vi "calcualte_Vr_Vi.vi"(5 "C2":fxp<+/-,32,3>=0.002117181196808815 format="%#_30g", 7 "C1":fxp<+/-,32,3>=0.9986428320407867 format="%#_31g", 8 "input valid":bool=TRUE, 9 "dw*dt":fxp<+/-,48,0>, 10 "Ii":fxp<+/-,16,14>, 11 "Ir":fxp<+/-,16,14>) -> (0 "output valid":bool, 2 "Vi":fxp<+/-,48,16>, 3 "Vr":fxp<+/-,48,16>)   [LabVIEW 2013]
uses:
  <vilib>/rvi/FXPMathLib/FxpMul/XNode/nifxpmath_Multiplier.xnode
  <vilib>/rvi/FXPMathLib/FxpAdd/XNode/nifxpmath_Add.xnode
  <vilib>/rvi/FXPMathLib/FxpSub/XNode/nifxpmath_Sub.xnode
  <vilib>/rvi/FXPMathLib/sim/FxpSim.dll
panel:
  # "1-w12*dt = 0.998643"
  # "Rl*w12*dt*(10^-9) = 0.0021171821211066989"
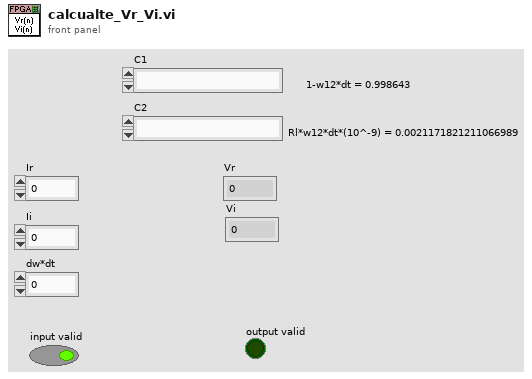
[diagram p1: front panel]
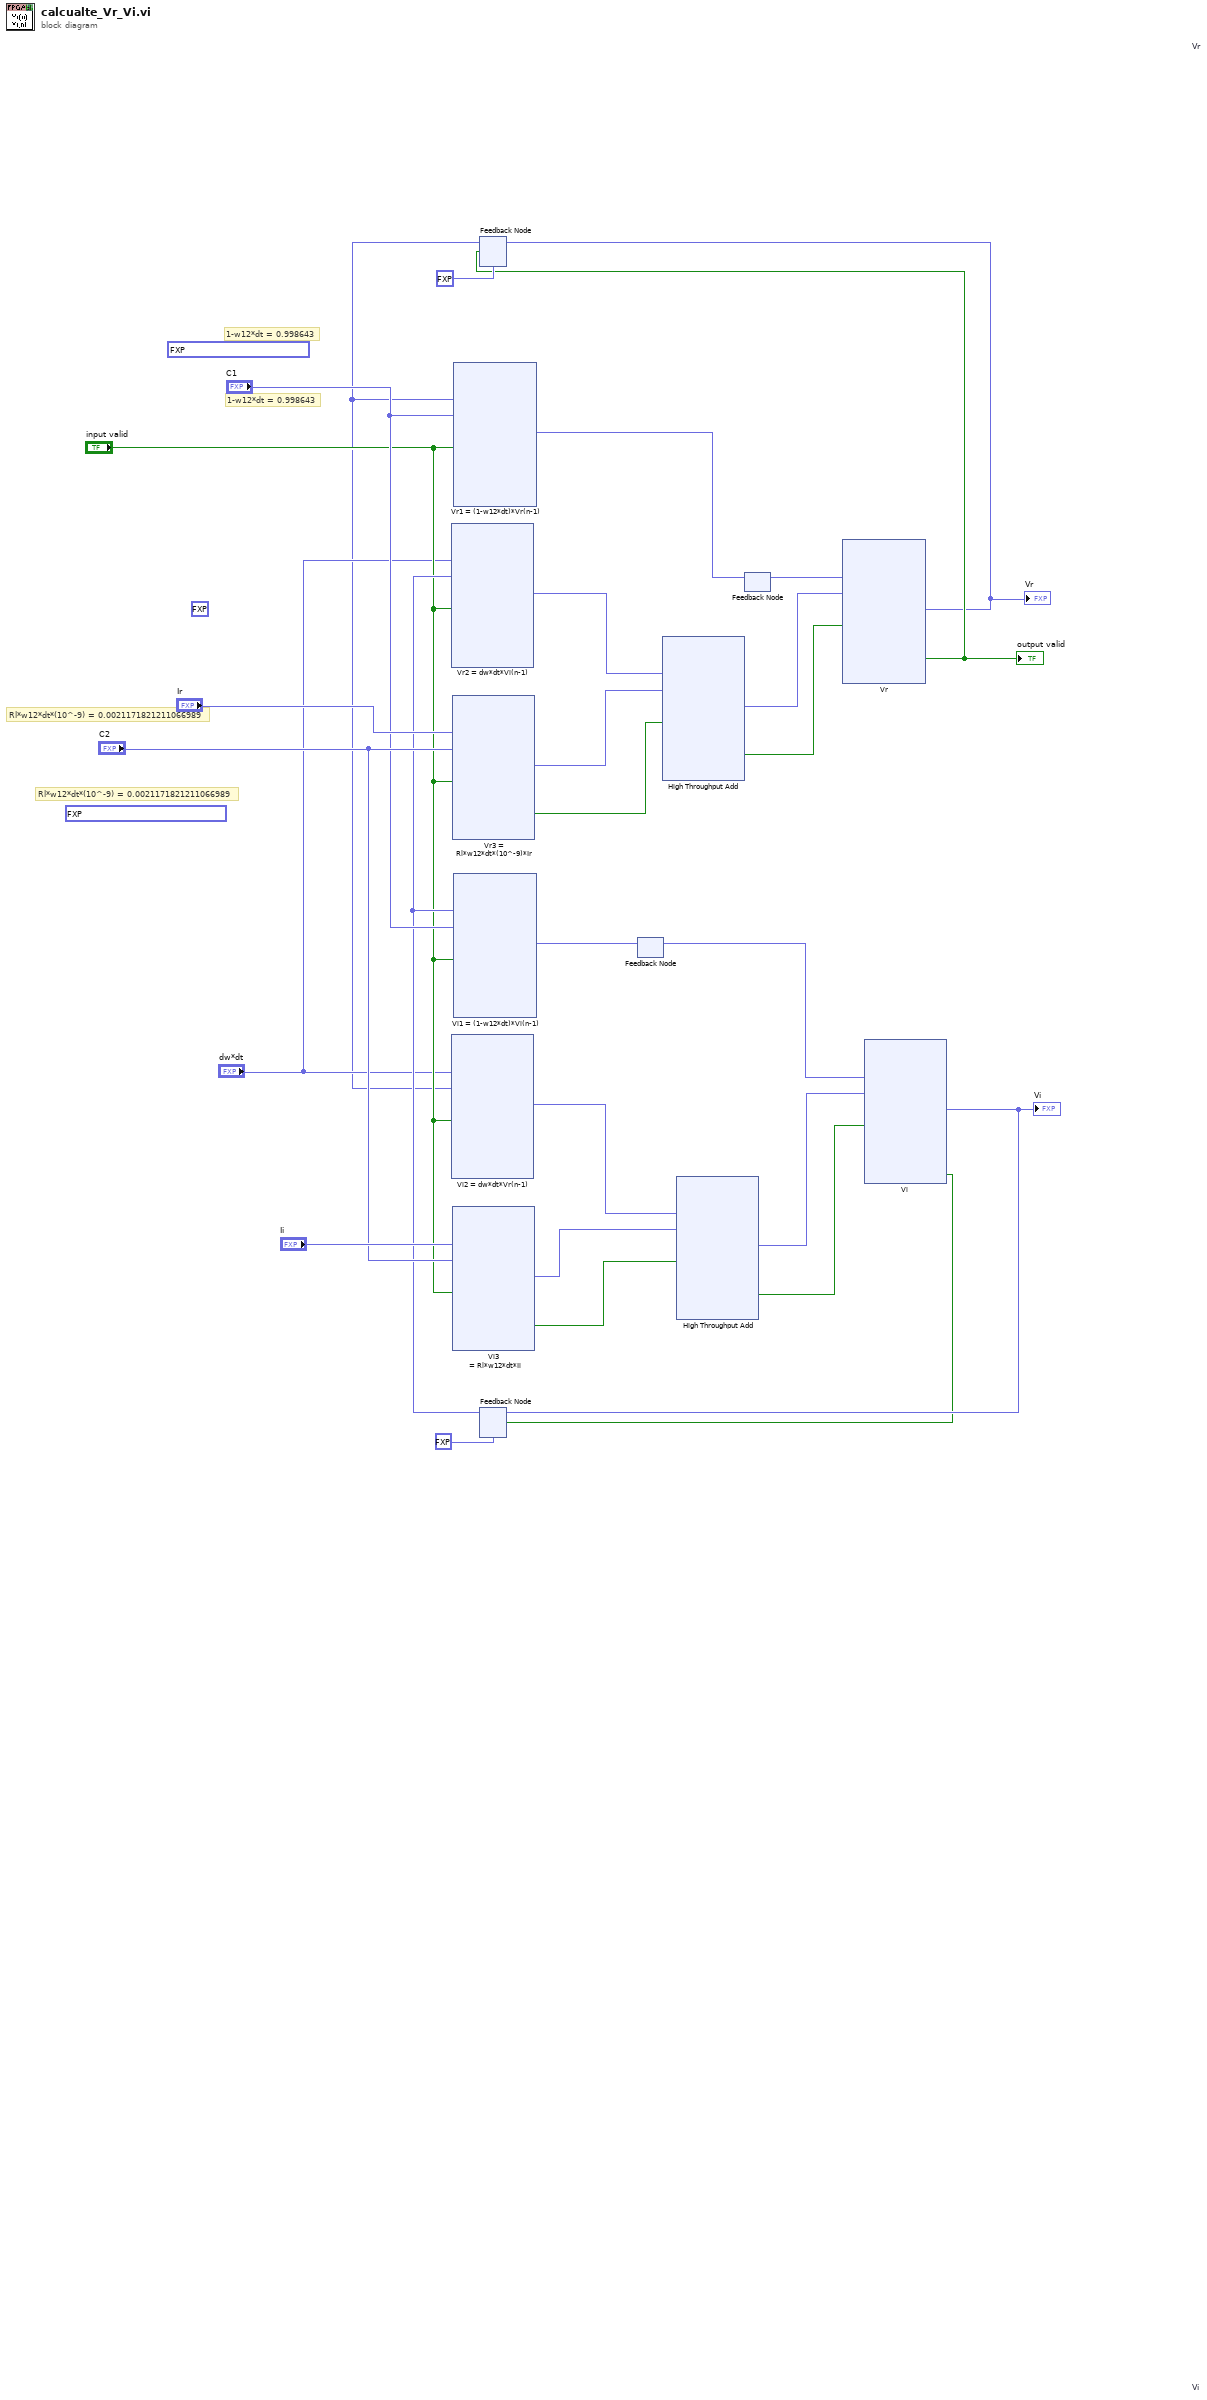
[diagram p0: block diagram]
diagram:
  (unwired) fxp<+/-,32,3> 0.0 ("x*y")
  (unwired) fxp<+/-,32,3> 0.002117181196808815 ("x")
  (unwired) fxp<+/-,32,3> 0.9986428320407867 ("x")
  # "Rl*w12*dt*(10^-9) = 0.0021171821211066989"
  # "1-w12*dt = 0.998643"
  # "Rl*w12*dt*(10^-9) = 0.0021171821211066989"
  # "1-w12*dt = 0.998643"
  n1 = xnode "Vr3 = Rl*w12*dt*(10^-9)*Ir"("x"="Ir", "y"="C2", "input valid"="input valid") -> ("x*y"=w13:fxp<+/-,32,6>, "output valid"=w12:bool)  [unwired: 1 in, 1 out]
  n2 = xnode "Vi3\n = Rl*w12*dt*Ii"("x"="Ii", "y"="C2", "input valid"="input valid") -> ("x*y"=w15:fxp<+/-,32,6>, "output valid"=w26:bool)  [unwired: 1 in, 1 out]
  n3 = feedback #1 "Vr"(fxp<+/-,48,16> 0.0 ("x+y")) -> (w3:fxp<+/-,48,16>)
  n4 = xnode "Vi2 = dw*dt*Vr(n-1)"("x"="dw*dt", "y"=w3, "input valid"="input valid") -> ("x*y"=w6:fxp<+/-,48,8>)  [unwired: 1 in, 2 out]
  n5 = xnode "Vr1 = (1-w12*dt)*Vr(n-1)"("x"=w3, "y"="C1", "input valid"="input valid") -> ("x*y"=w7:fxp<+/-,32,16>)  [unwired: 1 in, 2 out]
  n6 = feedback #2 "Vi"(fxp<+/-,48,16> 0.0 ("x+y")) -> (w19:fxp<+/-,48,16>)
  n7 = xnode "Vr2 = dw*dt*Vi(n-1)"("x"="dw*dt", "y"=w19, "input valid"="input valid") -> ("x*y"=w8:fxp<+/-,48,8>)  [unwired: 1 in, 2 out]
  n8 = xnode "Vi1 = (1-w12*dt)*Vi(n-1)"("x"=w19, "y"="C1", "input valid"="input valid") -> ("x*y"=w5:fxp<+/-,32,16>)  [unwired: 1 in, 2 out]
  n9 = feedback #3() -> (w24:fxp<+/-,32,16>)  [unwired: 1 in]
  n10 = feedback-in #3(w5) -> ()
  n11 = xnode ("High Throughput Add")("x"=w8, "y"=w13, "input valid"=w12) -> ("x+y"=w1:fxp<+/-,32,10>, "output valid"=w11:bool)  [unwired: 1 in, 1 out]
  n12 = xnode "High Throughput Add"("x"=w6, "y"=w15, "input valid"=w26) -> ("x+y"=w25:fxp<+/-,32,10>, "output valid"=w16:bool)  [unwired: 1 in, 1 out]
  n13 = feedback-in #4(w7) -> ()
  n14 = feedback #4() -> (w2:fxp<+/-,32,16>)  [unwired: 1 in]
  n15 = xnode "Vr"("x"=w2, "y"=w1, "input valid"=w11) -> ("x-y"=w9:fxp<+/-,48,16>, "output valid"=w10:bool)  [unwired: 1 in, 1 out]
  "Vr" <- w9
  "output valid" <- w10
  n16 = feedback-in #1(w9, w10) -> ()
  n17 = xnode "Vi"("x"=w24, "y"=w25, "input valid"=w16) -> ("x+y"=w18:fxp<+/-,48,16>, "ready for input"=w14:bool)  [unwired: 1 in, 1 out]
  "Vi" <- w18
  n18 = feedback-in #2(w18, w14) -> ()
